vi "Complete Manual.vi"(8 "error in (no error)":errorcluster, 10 "Model in":refnum<class "Model.lvclass">, 11 "Manual State in":refnum<class "Manual State.lvclass">) -> (0 "error out":errorcluster, 2 "Model out":refnum<class "Model.lvclass">, 3 "Manual State out":refnum<class "Manual State.lvclass">)   [LabVIEW 2016, in "Manual State.lvclass"]
uses:
  Manual State.lvclass
  Model/Model/Model.lvclass
  Typedefs/StateTypes.ctl
  Typedefs/HPMT_Typedefs.lvlib
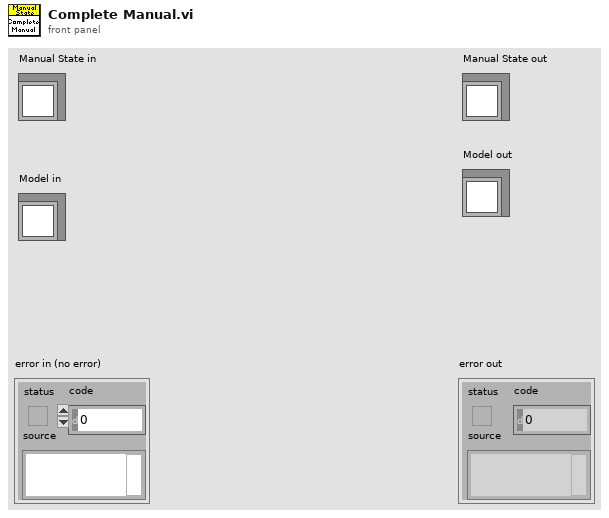
[diagram p1: front panel]
types:
  T1 = typedef "HPMT_Typedefs.lvlib/StateTypes.ctl" = enum16{"Offline State", "Fault State", "Standby State", "Disabled State", "Enabled State", "Wait For User Input State", "Test Actuator State", "Manual State"}
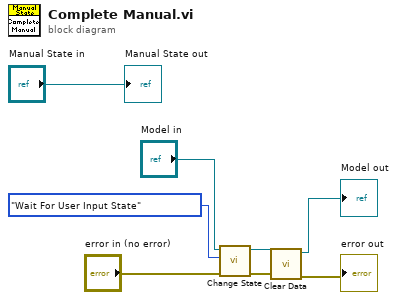
[diagram p0: block diagram]
diagram:
  n1 = call "Change State.vi"("error in (no error)"="error in (no error)", "State Types"=StateTypes."Wait For User Input State", "Model in"="Model in") -> ("error out"=w3:errorcluster, "Model out"=w4:refnum<class "Model.lvclass">)  [unwired: 7 in]
  n2 = call "Clear Data.vi"("error in (no error)"=w3, "Model in"=w4) -> ("error out"=→"error out":errorcluster, "Model out"=→"Model out":refnum<class "Model.lvclass">)  [unwired: 8 in]
  "Manual State out" <- "Manual State in"
